vi "NewtonsPSM_Meas_LCR.vi"(0 "VISA session":refnum<visa-resource-name>, 11 "error in (no error)":errorcluster) -> (4 "dup VISA session":refnum<visa-resource-name>, 6 "Read Strings":string, 8 "Measure":dbl[](array[numeric]) format="%^.4e", 15 "error out":errorcluster)   [LabVIEW 2025, in "NewtonsPSM1735.lvlib"]
doc: "This VI reads the LCR Data from the PPA2530."
uses:
  NewtonsPSM1735.lvlib
panel:
  # "Freq"
  # "Voltage"
  # "Current"
  # "Impedance"
  # "Phase"
  # "R series"
  # "L Series"
  # "C Series"
  # "R //"
  # "L //"
  # "C //"
  # "Tan d"
  # "Q Factor"
  # "Reactance"
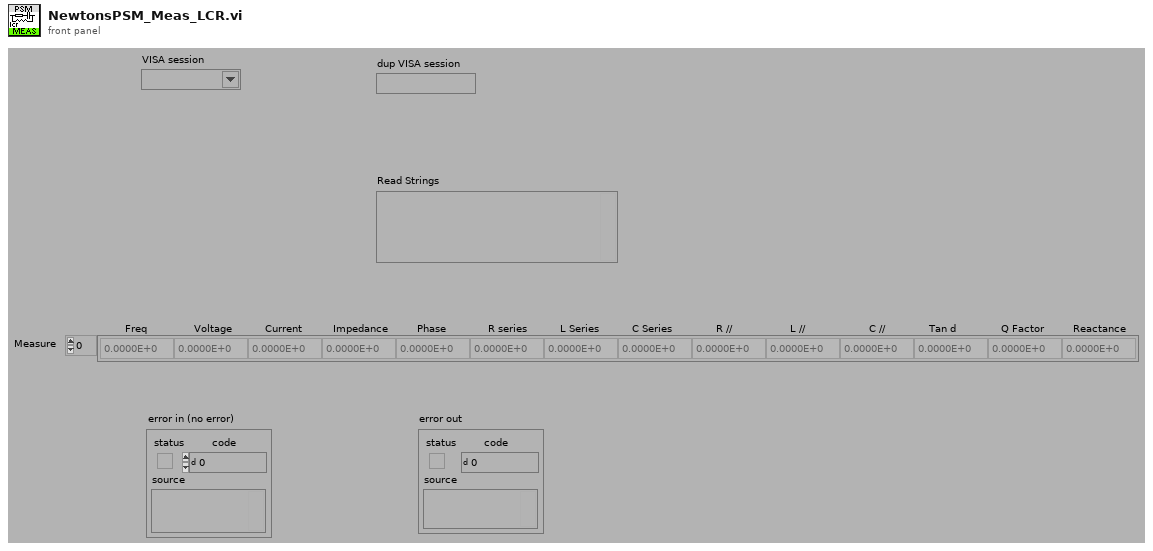
[diagram p1: front panel]
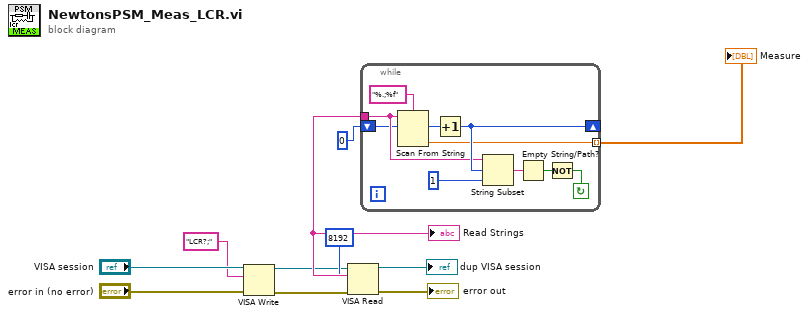
[diagram p0: block diagram]
diagram:
  n1 = VISA Write(VISA resource name="VISA session", write buffer="LCR?;", error in (no error)="error in (no error)") -> (VISA resource name out=w4:refnum<visa-resource-name>, error out=w3:errorcluster)  [unwired: 1 out]
  n2 = VISA Read(VISA resource name=w4, byte count=u32 8192 ("ÊÞ²Ä¶³ÝÄi0j"), error in (no error)=w3) -> (VISA resource name out=→"dup VISA session":refnum<visa-resource-name>, read buffer=w6:string, error out=→"error out":errorcluster)  [unwired: 1 out]
  "Read Strings" <- w6
  n3 = while {
    tunnel: [w13] -> w9 mode=indexing
    shift-left: 0 -> [w12]
    shift-right: [w17] -> _
    tunnel: w6 -> [w15]
    stop <- w18 continue-if-true
    n4 = Scan From String(format string="%.;%f", input string=w15, initial scan location=w12) -> (offset past scan=w14:u32, output 1=w13:dbl)  [unwired: 1 in, 3 out]
    n5 = Increment(x=w14) -> (x+1=w17:u32)
    n6 = String Subset(string=w15, offset (0)=w17, length (rest)=1) -> (substring=w20:string)
    n7 = Empty String/Path?(string/path=w20) -> (empty?=w19:bool)
    n8 = Not(x=w19) -> (.not. x?=w18:bool)
  }
  "Measure" <- w9
